vi "Read Load Settings.vi"(8 "error in (no error)":errorcluster, 11 "PacificPowerSource in":refnum<class "PacificPowerSource.lvclass">) -> (0 "error out":errorcluster, 2 "Load Settings":T1 {"Arbitrary Waveform"."Waveform Number (2: Arbitrary Waveform2)" items=["Arbitrary Waveform 2"=2, "Arbitrary Waveform 3"=3, "Arbitrary Waveform 4"=4, "Arbitrary Waveform 5"=5, "Arbitrary Waveform 6"=6, "Arbitrary Waveform 7"=7, "Arbitrary Waveform 8"=8, "Arbitrary Waveform 9"=9, "Arbitrary Waveform 10"=10, "Arbitrary Waveform 11"=11, "Arbitrary Waveform 12"=12, "Arbitrary Waveform 13"=13, "Arbitrary Waveform 14"=14, "Arbitrary Waveform 15"=15, "Arbitrary Waveform 16"=16, "Arbitrary Waveform 17"=17, "Arbitrary Waveform 18"=18, "Arbitrary Waveform 19"=19, "Arbitrary Waveform 20"=20, "Arbitrary Waveform 21"=21, "Arbitrary Waveform 22"=22]; "Waveform"."Waveform (1: Sine)" items=["Sine"=1, "Arbitrary Waveform 2"=2, "Arbitrary Waveform 3"=3, "Arbitrary Waveform 4"=4, "Arbitrary Waveform 5"=5, "Arbitrary Waveform 6"=6, "Arbitrary Waveform 7"=7, "Arbitrary Waveform 8"=8, "Arbitrary Waveform 9"=9, "Arbitrary Waveform 10"=10, "Arbitrary Waveform 11"=11, "Arbitrary Waveform 12"=12, "Arbitrary Waveform 13"=13, "Arbitrary Waveform 14"=14, "Arbitrary Waveform 15"=15, "Arbitrary Waveform 16"=16, "Arbitrary Waveform 17"=17, "Arbitrary Waveform 18"=18, "Arbitrary Waveform 19"=19, "Arbitrary Waveform 20"=20, "Arbitrary Waveform 21"=21, "Arbitrary Waveform 22"=22]; "Waveform"."Channel Name (1: A)" items=["A"=1, "B"=2, "C"=3]; "Frequency"."Frequency Range (600Hz)" items=["150 Hz", "300 Hz", "600 Hz", "1200 Hz"]; "Range Control (0: Auto)" items=["Auto", "<110 V", "110 V -120.9 V", "121 V - 130.9 V", "> 131 V"]; "Configure Output"."Form (3: Three)" items=["Single", "Split", "Three"]; "Configure Output"."Coupling  (0: Direct)" items=["Direct", "Transformer"]}, 3 "PacificPowerSource out":refnum<class "PacificPowerSource.lvclass">)   [LabVIEW 2018, in "AcPwrPlugins.lvlib" / "PacificPowerSource.lvclass"]
uses:
  PacificPowerSource.lvclass
  TypeDefs/DeviceSettings.ctl
  PacificPowerSource.lvclass/PacificPowerSource.ctl
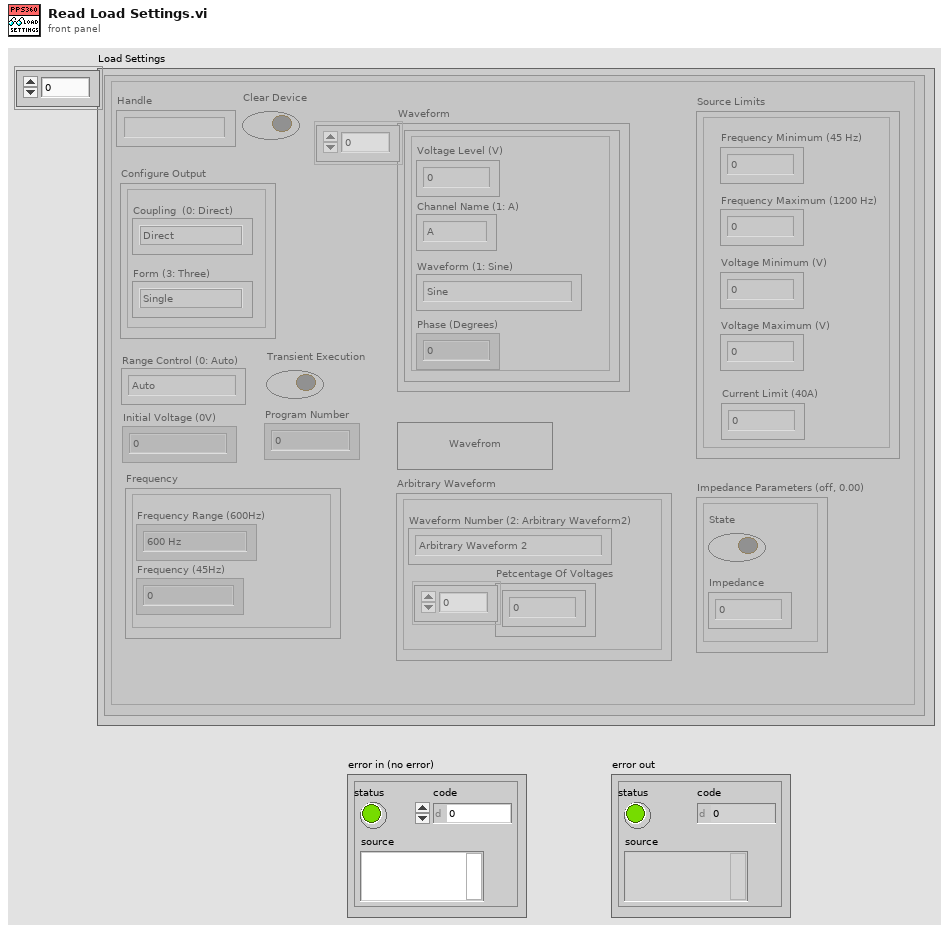
[diagram p1: front panel]
types:
  T1 = typedef "AcPwrPlugins.lvlib/PacificPowerSource.lvclass/DeviceSettings.ctl" = cluster{"Handle":string, "Connected":bool, "Source Limits":cluster{"Frequency Minimum (45 Hz)":dbl, "Frequency Maximum (1200 Hz)":dbl, "Voltage Maximum (V)":dbl, "Voltage Minimum (V)":dbl, "Current Limit (40A)":dbl}, "Clear Device":bool, "Configure Output":cluster{"Coupling  (0: Direct)":u16, "Form (3: Three)":u16}, "Range Control (0: Auto)":u16, "Initial Voltage (0V)":u16, "Frequency":cluster{"Frequency Range (600Hz)":u16, "Frequency (45Hz)":dbl}, "Waveform":cluster{"Voltage Level (V)":dbl, "Phase (Degrees)":i32, "Channel Name (1: A)":u16, "Waveform (1: Sine)":u16}[], "Arbitrary Waveform":cluster{"Waveform Number (2: Arbitrary Waveform2)":u16, "Petcentage Of Voltages":dbl[]}, "Impedance Parameters (off, 0.00)":cluster{"State":bool, "Impedance":dbl}, "Waveform Type":bool, "Program Number":i32, "Transient Execution":bool}[]
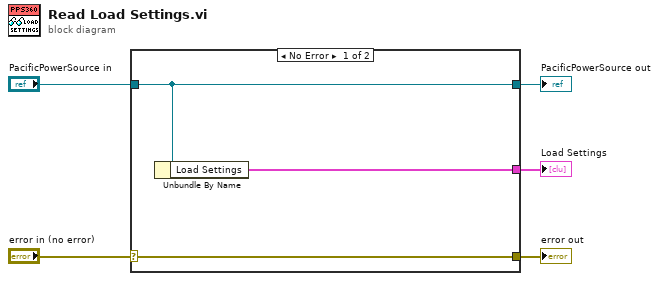
[diagram p0: block diagram]
diagram:
  n1 = case shown="No Error" "error in (no error)" {
    selector: "error in (no error)" -> [w8 w9]
    tunnel: [w8 w9] -> w4
    tunnel: [w7 w10] -> w2
    tunnel: "PacificPowerSource in" -> [w7 w10]
    tunnel: [w6 _] -> w1
    frame No Error {
      n2 = Unbundle By Name(w7) -> ("Load Settings"=w6:T1)
    }
    frame Error {
    }
  }
  "error out" <- w4
  "PacificPowerSource out" <- w2
  "Load Settings" <- w1
